vi "ShapeDetection Circle.vi"(0 "Image Dst In":T3, 1 "ParameterIn":T1={"Curve Parameters"={"Extraction Mode"=enum."Normal", "Edge Threshold"=75, "Edge Filter Size"=enum."Normal", "Min Length"=25, "Row Search Step Size"=15, "Col Search Step Size"=15, "Max Endpoint Gap"=10, "Closed"=FALSE, "Subpixel"=FALSE}, "Circle Descriptor"={"Min Radius"=3.0, "Max Radius"=500.0}, "Match Options"={"Rotation"=TRUE, "Scale"=FALSE, "Occlusion"=FALSE, "Range Settings"=[]}, "Minimum match score"=800.0, "SetCircleNum"=0}, 2 "ROI Descriptor":T2={"Global Rectangle"=[20, 20, 1260, 1004], "Contours"=[{"ID"=enum."External", "Type"=3, "Coordinates"=[20, 20, 1260, 1004]}]} {"Contours"."Type" items=["No Selection", "Point", "Line", "Rectangle", "Oval", "Polygon", "Freehand Region", "Annulus", "Unused2", "Unused3", "Broken Line", "Freehand Line", "Rotated Rectangle"]}, 5 "error in":errorcluster) -> (14 "Image Out":T3(plugin-control), 15 "Circles":T4(array[cluster]), 16 "Str_Result":string, 17 "Numbers":i32, 19 "error out":errorcluster)   [LabVIEW 2019]
uses:
  <vilib>/vision/NI_Vision_Development_Module.lvlib
  <vilib>/vision/Image Controls.llb/IMAQ Image.ctl
panel:
  in  "errorIn":errorcluster
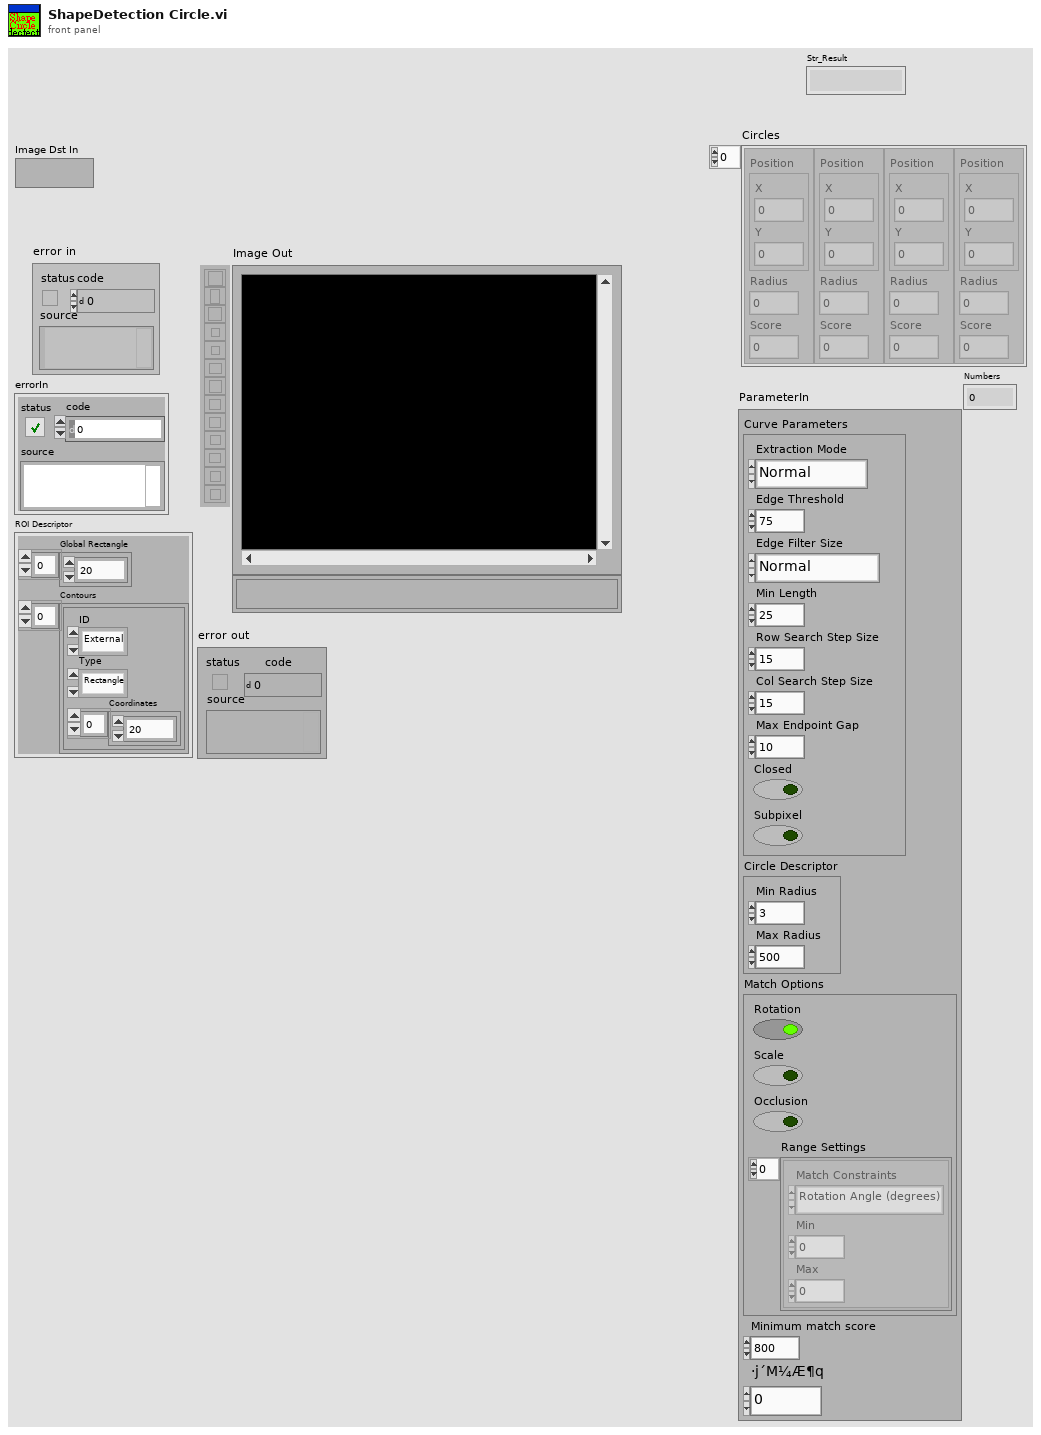
[diagram p1: front panel]
types:
  T1 = cluster{"Curve Parameters":cluster{"Extraction Mode":enum16{"Normal", "Uniform Regions"}, "Edge Threshold":i32, "Edge Filter Size":enum16{"Fine", "Normal"}, "Min Length":i32, "Row Search Step Size":i32, "Col Search Step Size":i32, "Max Endpoint Gap":i32, "Closed":bool, "Subpixel":bool}, "Circle Descriptor":cluster{"Min Radius":dbl, "Max Radius":dbl}, "Match Options":cluster{"Rotation":bool, "Scale":bool, "Occlusion":bool, "Range Settings":cluster{"Match Constraints":enum16{"Rotation Angle (degrees)", "Scale Factor (%)", "Occlusion (%)"}, "Min":dbl, "Max":dbl}[]}, "Minimum match score":dbl, "SetCircleNum":i32}
  T2 = cluster{"Global Rectangle":i32[], "Contours":cluster{"ID":enum32{"External", "Internal"}, "Type":u32, "Coordinates":i32[]}[]}
  T3 = typedef "IMAQ Image.ctl" = refnum<image>
  T4 = cluster{"Position":cluster{"X":sgl, "Y":sgl}, "Radius":dbl, "Score":dbl}[]
  T5 = typedef "Image Type" = u32
  T6 = cluster{"histogram":u32[], "Minimal Value":sgl, "Maximal Value":sgl, "Starting Value":sgl, "Interval Width":sgl, "Mean Value":sgl, "Standard  Variation":sgl, "Area (pixels)":i32}
  T7 = cluster{"Extraction Mode":enum16{"Normal", "Uniform Regions"}, "Edge Threshold":i32, "Edge Filter Size":enum16{"Fine", "Normal"}, "Min Length":i32, "Row Search Step Size":i32, "Col Search Step Size":i32, "Max Endpoint Gap":i32, "Closed":bool, "Subpixel":bool}
  T8 = cluster{"Rotation":bool, "Scale":bool, "Occlusion":bool, "Range Settings":cluster{"Match Constraints":enum16{"Rotation Angle (degrees)", "Scale Factor (%)", "Occlusion (%)"}, "Min":dbl, "Max":dbl}[]}
  T9 = cluster{"Position":cluster{"X":sgl, "Y":sgl}, "Radius":dbl, "Score":dbl}
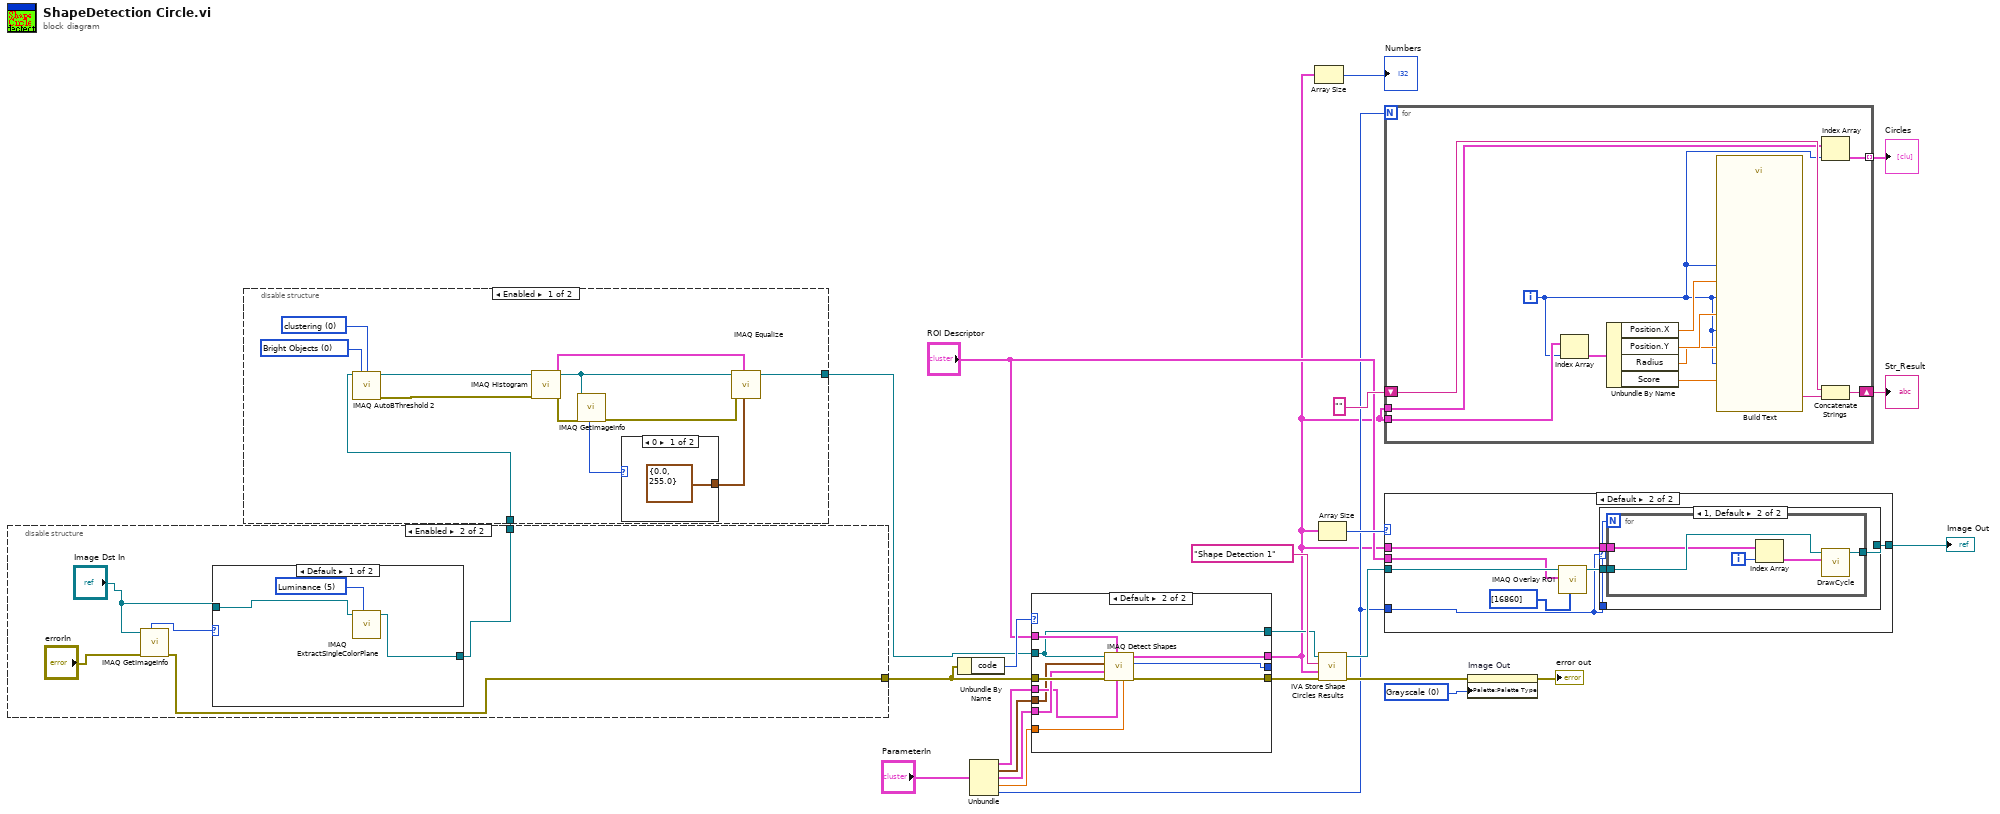
[diagram p0: block diagram]
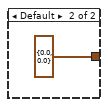
[diagram p2: hidden frame]
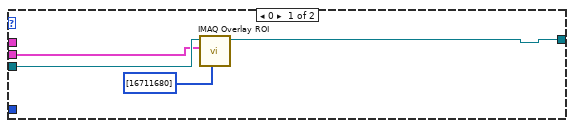
[diagram p4: hidden frame]
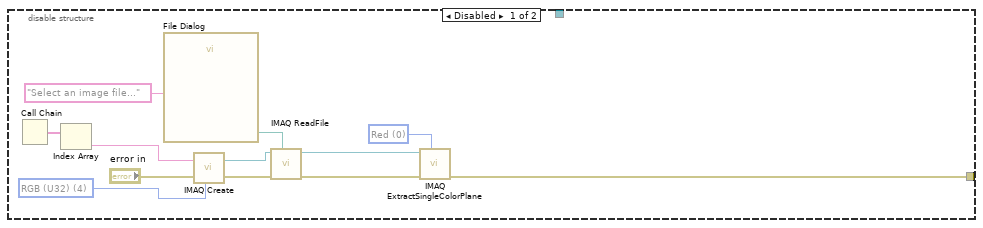
[diagram p6: hidden frame]
diagram:
  w20 = u32 0 items=["Grayscale", "Binary", "Gradient", "Rainbow", "Temperature", "User Defined"] ("Palette")
  n1 = disable-structure shown="Enabled" {
    disable-tunnel: [w27 w40] -> w25
    disable-tunnel: [_ w39] -> w2
    frame Disabled {
      w29 = 0 items=["Red", "Green", "Blue", "Hue", "Saturation", "Luminance", "Value", "Intensity"] ("Color Plane")
      w30 = T5 4 items=["Grayscale (U8)", "Grayscale (I16)", "Grayscale (SGL)", "Complex (CSG)", "RGB (U32)", "HSL (U32)", "RGB (U64)", "Grayscale (U16)"] ("Image Type")
      n2 = Call Chain() -> (call chain=w34:string[])
      n3 = Index Array(array=w34) -> (element=w33:string)  [unwired: 1 in]
      n4 = call "File Dialog"("prompt"="Select an image file...") -> ("selected path"=w31:path)  [unwired: 6 in, 8 out]
      n5 = call "IMAQ Create"("Image Name"=w33, "Image Type"=w30, "error in (no error)"="error in") -> ("New Image"=w37:T3, "error out"=w36:errorcluster)  [unwired: 1 in, 1 out]
      n6 = call "IMAQ ReadFile"("File Path"=w31, "error in (no error)"=w36, "Image"=w37) -> ("error out"=w38:errorcluster, "Image Out"=w28:T3)  [unwired: 2 in, 5 out]
      n7 = call "IMAQ ExtractSingleColorPlane"("Color Plane"=w29, "error in (no error)"=w38, "Image Src"=w28) -> ("error out"=w27:errorcluster, "Image Dst Out"=w26:T3)  [unwired: 1 in, 6 out]
    }
    frame Enabled {
      n8 = call "IMAQ GetImageInfo"("error in (no error)"="errorIn", "Image"="Image Dst In") -> ("error out"=w40:errorcluster, "Image Type"=w43:T5)  [unwired: 2 in, 6 out]
      n9 = case shown="Default" w43 {
        tunnel: "Image Dst In" -> [w46 w47]
        tunnel: [w44 w47] -> w39
        frame Default {
          w45 = 5 items=["Red", "Green", "Blue", "Hue", "Saturation", "Luminance", "Value", "Intensity"] ("Color Plane")
          n10 = call "IMAQ ExtractSingleColorPlane"("Color Plane"=w45, "Image Src"=w46) -> ("Image Dst Out"=w44:T3)  [unwired: 8 in, 1 out]
        }
        frame 0 {
        }
      }
    }
  }
  n11 = disable-structure shown="Enabled" {
    disable-tunnel: w2 -> [w49 w61]
    disable-tunnel: [w48 w61] -> w1
    frame Enabled {
      w52 = 0 items=["clustering", "entropy", "metric", "moments", "inter-class variance"] ("Method")
      w51 = u32 0 items=["Bright Objects", "Dark Objects"] ("Look For")
      n12 = call "IMAQ AutoBThreshold 2"("Image Src"=w49, "Look For (Bright Objects)"=w51, "Method (clustering)"=w52) -> ("Image Dst Out"=w55:T3, "error out"=w50:errorcluster)  [unwired: 5 in, 6 out]
      n13 = call "IMAQ Histogram"("error in (no error)"=w50, "Image"=w55) -> ("error out"=w56:errorcluster, "Histogram Report"=w53:T6)  [unwired: 3 in, 5 out]
      n14 = call "IMAQ GetImageInfo"("error in (no error)"=w56, "Image"=w55) -> ("error out"=w57:errorcluster, "Image Type"=w54:T5)  [unwired: 8 out]
      n15 = case shown="0" w54 {
        tunnel: [cluster{"Minimum":sgl, "Maximum":sgl} {"Minimum"=0.0, "Maximum"=255.0} ("Range") cluster{"Minimum":sgl, "Maximum":sgl} {"Minimum"=0.0, "Maximum"=0.0} ("Range")] -> w58
        frame 0 {
        }
        frame Default {
        }
      }
      n16 = call "IMAQ Equalize"("Range"=w58, "Histogram Report"=w53, "error in (no error)"=w57, "Image Src"=w55) -> ("Image Dst Out"=w48:T3)  [unwired: 2 in, 5 out]
    }
    frame Disabled {
    }
  }
  n17 = Unbundle By Name(w25) -> ("code"=w22:i32)
  n18 = Unbundle("ParameterIn") -> ("Curve Parameters"=w13:T7, "Circle Descriptor"=w15:cluster{"Min Radius":dbl, "Max Radius":dbl}, "Match Options"=w14:T8, "Minimum match score"=w12:dbl, "SetCircleNum"=w4:i32)
  n19 = case shown="Default" w22 {
    tunnel: w25 -> [_ w72]
    tunnel: [_ w71] -> _
    tunnel: w14 -> [_ w70]
    tunnel: w13 -> [_ w69]
    tunnel: w12 -> [_ w68]
    tunnel: w15 -> [_ w67]
    tunnel: "ROI Descriptor" -> [_ w66]
    tunnel: [_ w65] -> w3
    tunnel: w1 -> [w62 w63]
    tunnel: [_ w64] -> w24
    tunnel: [w62 w63] -> w21
    frame -1074396199, -1074396198 {
      # "Discard Coordinate\nSystem Error"
    }
    frame Default {
      n20 = call-poly "IMAQ Detect Shapes"("Minimum match score"=w68, "Curve Parameters"=w69, "ROI Descriptor"=w66, "error in (no error)"=w72, "Match Options"=w70, "Circle Descriptor"=w67, "Image"=w63) -> ("error out"=w64:errorcluster, "Number of Matches Returned"=w71:i32, "Circles"=w65:T4)  [unwired: 2 out]
    }
  }
  n21 = Array Size(array=w3) -> (size(s)=→"Numbers":i32)
  n22 = Array Size(array=w3) -> (size(s)=w7:i32)
  n23 = call <vilib>:"IVA Store Shape Circles Results.vi"("error in (no error)"=w24, "Circles"=w3, "Step Name"="Shape Detection 1", "Image in"=w21) -> ("error out"=w9:errorcluster, "Image dup"=w11:T3)  [unwired: 6 out]
  n24 = for {
    N: w4 -> [_]
    tunnel: w3 -> [w84]
    shift-right: [w78] -> w17
    shift-left: "" -> [w77]
    tunnel: w3 -> [w75]
    tunnel: [w74] -> w5 mode=indexing
    i -> [w73]
    n25 = Index Array(array=w84, index=w73) -> (element=w76:T9)
    n26 = Unbundle By Name(w76) -> ("Position.X"=w83:sgl, "Position.Y"=w82:sgl, "Radius"=w81:dbl, "Score"=w80:dbl)
    n27 = call "Build Text"("Posy"=w82, "Radius"=w81, "Score"=w80, "Ind"=w73, "Posx"=w83, "Ind2"=w73, "Ind3"=w73, "Ind4"=w73) -> ("Result"=w79:string)  [unwired: 6 in, 1 out]
    n28 = Index Array(array=w75, index=w73) -> (element=w74:T9)
    n29 = Concatenate Strings(w77, w79) -> (w78:string)
  }
  "Circles" <- w5
  "Str_Result" <- w17
  n30 = case shown="Default" w7 {
    tunnel: w11 -> [w88 w95]
    tunnel: [w85 w94] -> w10
    tunnel: w3 -> [_ w93]
    tunnel: "ROI Descriptor" -> [w86 w91]
    tunnel: w4 -> [_ w89]
    frame 0 {
      n31 = call "IMAQ Overlay ROI"("Colors (Green)"=u32[] [16711680], "ROI Descriptor"=w86, "Image"=w88) -> ("Image Out"=w85:T3)  [unwired: 7 in, 1 out]
    }
    frame Default {
      n32 = call "IMAQ Overlay ROI"("Colors (Green)"=u32[] [16860], "ROI Descriptor"=w91, "Image"=w95) -> ("Image Out"=w92:T3)  [unwired: 7 in, 1 out]
      n33 = case shown="1, Default" w89 {
        tunnel: [w96 w100] -> w94
        tunnel: w93 -> [_ w99]
        tunnel: w92 -> [w96 w98]
        tunnel: w89 -> [_ w97]
        frame 0 {
        }
        frame 1, Default {
          n34 = for {
            N: w97 -> [_]
            tunnel: w98 -> [w105]
            tunnel: [w104] -> w100
            tunnel: w99 -> [w103]
            i -> [w101]
            n35 = Index Array(array=w103, index=w101) -> (element=w102:T9)
            n36 = call "DrawCycle.vi"("CirclesDataIn"=w102, "ImageIn"=w105) -> ("Image Out"=w104:T3)  [unwired: 9 in]
          }
        }
      }
    }
  }
  "Image Out" <- w10
  n37 = property on="Image Out" class="ImageControl"(error in=w9, "Palette:Palette Type"=w20) -> (error out=→"error out":errorcluster)  [unwired: 1 in, 1 out]
